vi "Untitled 1.vi"() -> ()   [LabVIEW 2014]
panel:
  in  "switch_control_array":T1(array[cluster])=[{"switch_posit"={"x"=0.0, "y"=0.0, "z"=0.0}, "switch"=FALSE, "invert"=FALSE, "wait"=0.0}]
  in  "switch_data_array":T2(array[cluster])=[{"switch_posit"={"x"=0.0, "y"=0.0, "z"=0.0}, "manual"=FALSE}]
  in  "train_control_array":T3(array[cluster])=[{"uuid"="uuid", "throttle"=0.0, "brake"=0.0, "horn"=0.0, "wait"=0.0, "name"="", "mode"="", "dest"=""}]
  in  "train_data_array":T4(array[cluster])=[{"uuid"="uuid", "int"=0, "posit_array"=[{"x"=0.0, "y"=0.0, "z"=0.0}, {"x"=1.0, "y"=1.0, "z"=1.0}]}]
  out "JSON string 5":string
  out "JSON string 4":string
  out "JSON string 3":string
  out "JSON string 2":string
  out "JSON string":string
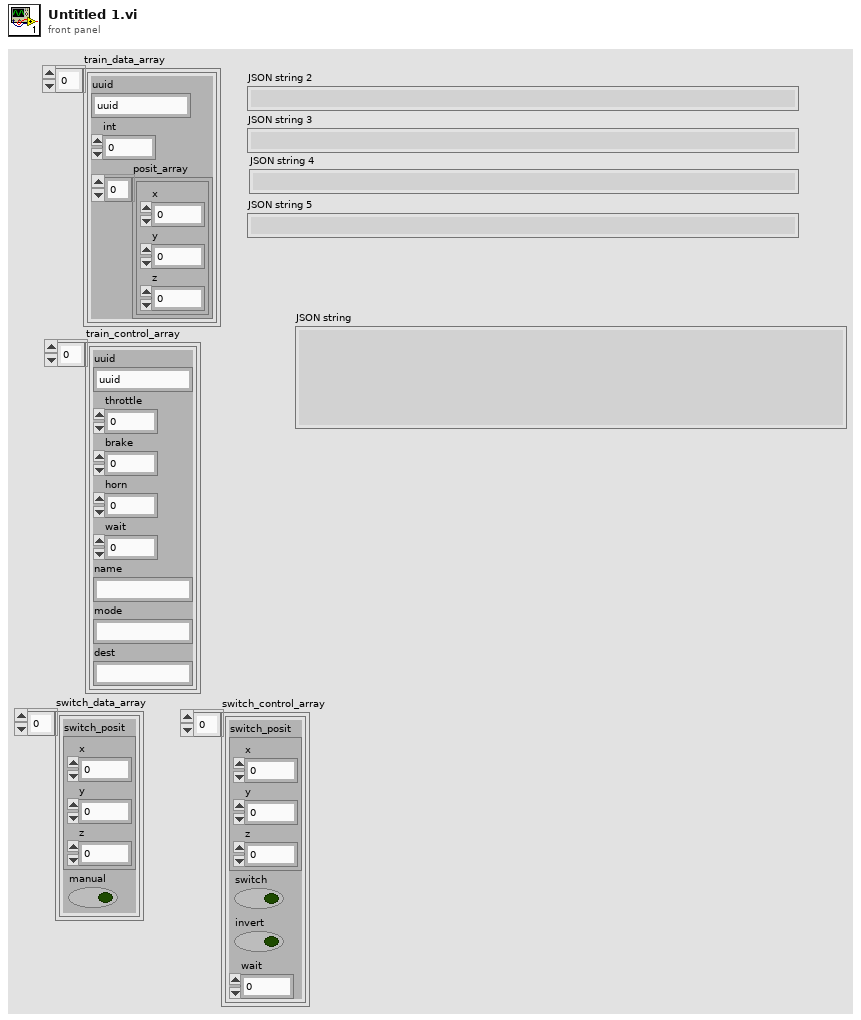
[diagram p1: front panel]
types:
  T1 = cluster{"switch_posit":cluster{"x":dbl, "y":dbl, "z":dbl}, "switch":bool, "invert":bool, "wait":dbl}[]
  T2 = cluster{"switch_posit":cluster{"x":dbl, "y":dbl, "z":dbl}, "manual":bool}[]
  T3 = cluster{"uuid":string, "throttle":dbl, "brake":dbl, "horn":dbl, "wait":dbl, "name":string, "mode":string, "dest":string}[]
  T4 = cluster{"uuid":string, "int":i32, "posit_array":cluster{"x":dbl, "y":dbl, "z":dbl}[]}[]
  T5 = cluster{"train_data_array":cluster{"uuid":string, "int":i32, "posit_array":cluster{"x":dbl, "y":dbl, "z":dbl}[]}[], "train_control_array":cluster{"uuid":string, "throttle":dbl, "brake":dbl, "horn":dbl, "wait":dbl, "name":string, "mode":string, "dest":string}[], "switch_data_array":cluster{"switch_posit":cluster{"x":dbl, "y":dbl, "z":dbl}, "manual":bool}[], "switch_control_array":cluster{"switch_posit":cluster{"x":dbl, "y":dbl, "z":dbl}, "switch":bool, "invert":bool, "wait":dbl}[]}
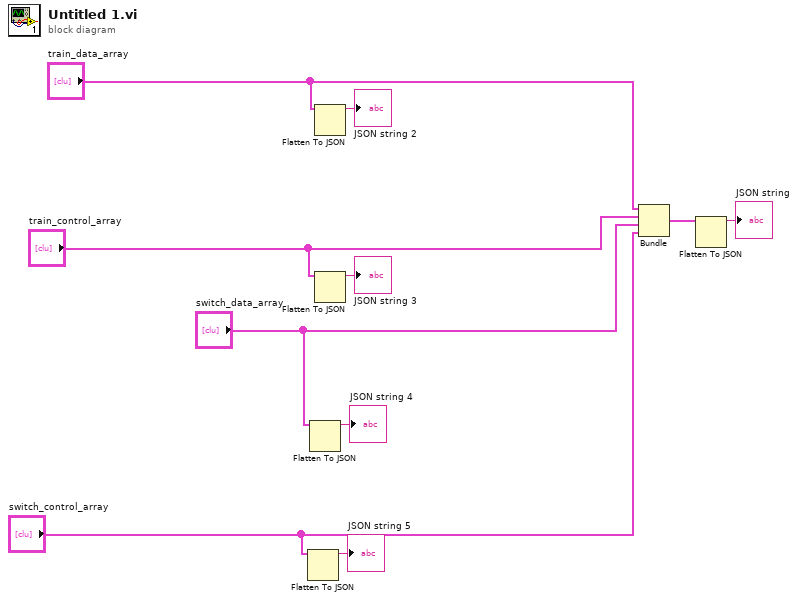
[diagram p0: block diagram]
diagram:
  n1 = Flatten To JSON(anything="switch_control_array") -> (JSON string=→"JSON string 5":string)  [unwired: 2 in, 1 out]
  n2 = Flatten To JSON(anything="switch_data_array") -> (JSON string=→"JSON string 4":string)  [unwired: 2 in, 1 out]
  n3 = Flatten To JSON(anything="train_data_array") -> (JSON string=→"JSON string 2":string)  [unwired: 2 in, 1 out]
  n4 = Flatten To JSON(anything="train_control_array") -> (JSON string=→"JSON string 3":string)  [unwired: 2 in, 1 out]
  n5 = Bundle("train_data_array"="train_data_array", "train_control_array"="train_control_array", "switch_data_array"="switch_data_array", "switch_control_array"="switch_control_array") -> (w10:T5)  [unwired: 1 in]
  n6 = Flatten To JSON(anything=w10) -> (JSON string=→"JSON string":string)  [unwired: 2 in, 1 out]
